vi "labview3.vi"() -> ()   [LabVIEW 2015]
panel:
  out "?":dbl
  out "Boolean 2":bool
  in  "km/h":dbl
  in  "Boolean":bool
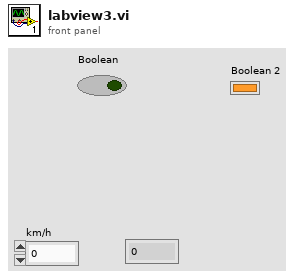
[diagram p1: front panel]
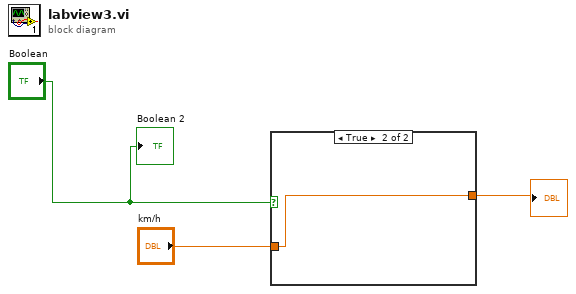
[diagram p0: block diagram]
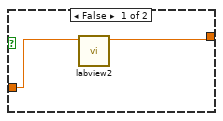
[diagram p2: hidden frame]
diagram:
  n1 = case shown="True" "Boolean" {
    tunnel: "km/h" -> [w5 w6]
    tunnel: [w4 w6] -> w1
    frame False {
      n2 = call "labview2.vi"("km/h"=w5) -> ("ms/s"=w4:dbl)  [unwired: 10 in]
    }
    frame True {
    }
  }
  "?" <- w1
  "Boolean 2" <- "Boolean"
